vi "Initialize.vi"(2 "error in":errorcluster) -> (0 "error out":errorcluster, 1 "Enum":T1(ring)=enum."Execute")   [LabVIEW 2017]
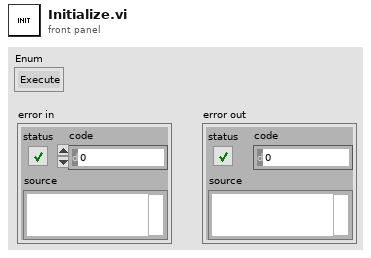
[diagram p1: front panel]
types:
  T1 = enum16{"Terminate", "Finalize", "Execute", "Initialize"}
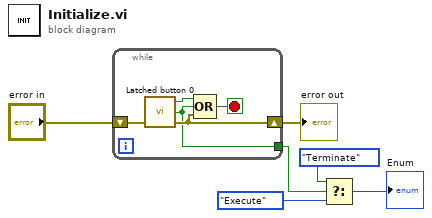
[diagram p0: block diagram]
diagram:
  n1 = while {
    shift-right: [w10] -> w4
    shift-left: "error in" -> [w11]
    tunnel: [w7] -> w5
    stop <- w8 stop-if-true
    n2 = call "Latched button 0.vi"("error in (no error)"=w11) -> ("error out"=w10:errorcluster, "Long Pressed"=w7:bool, "Latched"=w9:bool)  [unwired: 2 in]
    n3 = Compound Arithmetic op=OR(w9, w7, w10) -> (w8:bool)
  }
  "error out" <- w4
  n4 = Select(t=T1."Terminate", s=w5, f=T1."Execute") -> (s? t:f=→"Enum":T1)
